vi "Autonomous Independent.vi"() -> ()   [LabVIEW 2019]
doc: "This VI is called when autonomous begins, and will automatically be terminated when autonomous ends. You can carry out timed or sensor driven robot movement independently without needing to return to the caller."
uses:
  Robot Global Data.vi
  <vilib>/Rock Robotics/Network Tables/SD Write Boolean.vi
panel:
  in  "v scale":dbl=1.0
  # "Be sure to right-click and choose Data Operations>>Make Current Value default if you want to save the array values with the VI"
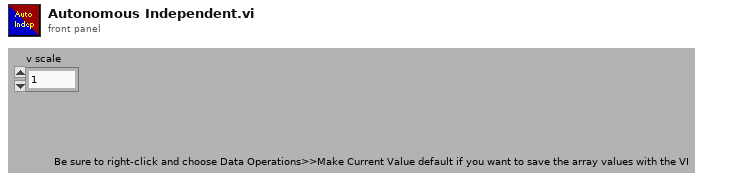
[diagram p1: front panel]
types:
  T1 = typedef "WPI_JoystickDevRef.ctl" = cluster{"Device":T2}
  T2 = typedef "WPI_JoystickDeviceEnum.ctl" = enum16{"USB 0", "USB 1", "USB 2", "USB 3", "USB 4", "USB 5"}
  T3 = cluster{"Cluster":cluster{"Path Backwards":bool, "Robot Backwards":bool}, "Traj Vel Points":cluster{"V":dbl, "th":dbl}[], cluster{"Sample Period (s)":dbl, cluster{"Velocity (fps)":dbl, "Acceleration (fps^2)":dbl, "Jerk (fps^3)":dbl, dbl}, "Conditions":cluster{"vInitial (fps)":dbl, "vFinal (fps)":dbl}, "Angular Accelerations":cluster{"Angular \nAccelerations":dbl[], "Override Limits?":bool[]}}}[]
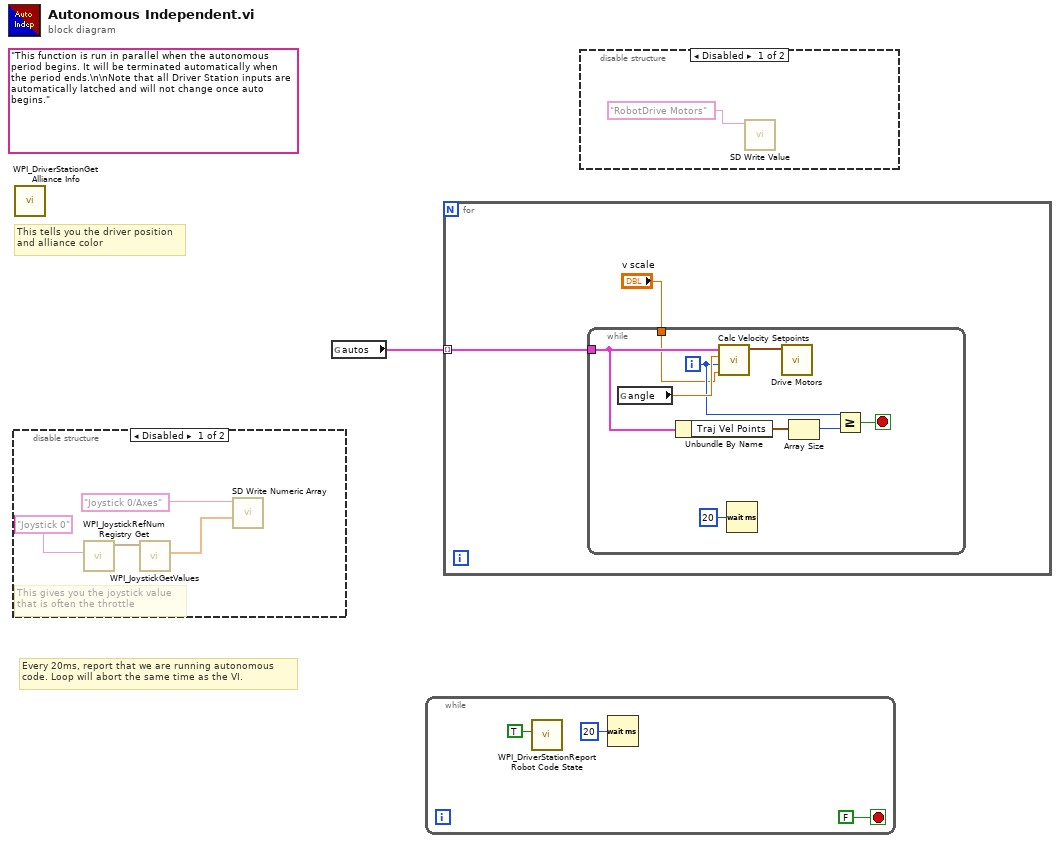
[diagram p0: block diagram]
diagram:
  (unwired) "This function is run in parallel when the autonomous period begins. It will be terminated automatically when the period ends.\n\nNote that all Driver Station inputs are automatically latched and will not change once auto begins."
  # "Every 20ms, report that we are running autonomous\ncode. Loop will abort the same time as the VI."
  # "This tells you the driver position\nand alliance color"
  n1 = disable-structure shown="Disabled" {
    frame Disabled {
      # "This gives you the joystick value\nthat is often the throttle"
      n2 = call <vilib>:"WPI_JoystickRefNum Registry Get.vi"("refnum name"="Joystick 0") -> ("JoystickDevRef"=w4:T1)  [unwired: 1 in, 9 out]
      n3 = call <vilib>:"WPI_JoystickGetValues.vi"("JoystickDevRef"=w4) -> ("Axes"=w2:dbl[])  [unwired: 6 in, 4 out]
      n4 = call <vilib>:"SD Write Numeric Array.vi"("Numeric Array"=w2, "Name"="Joystick 0/Axes") -> ()  [unwired: 8 in, 2 out]
    }
    frame Enabled {
    }
  }
  n5 = call <vilib>:"WPI_DriverStationGet Alliance Info.vi"() -> ()  [unwired: 12 out]
  n6 = global read "Robot Global Data.vi" "autos"() -> (w1:T3)
  n7 = while {
    stop <- FALSE stop-if-true
    n8 = call <vilib>:"WPI_DriverStationReport Robot Code State.vi"("Autonomous"=TRUE) -> ()  [unwired: 10 in, 1 out]
    n9 = Wait (ms)(milliseconds to wait=u32 20) -> ()  [unwired: 1 out]
  }
  n10 = for {
    tunnel: w1 -> [w10] mode=indexing
    n11 = while {
      tunnel: w10 -> [w16]
      tunnel: "v scale" -> [w11]
      i -> [w13]
      stop <- w12 stop-if-true
      n12 = global read "Robot Global Data.vi" "angle"() -> (w18:dbl)
      n13 = Unbundle By Name(w16) -> ("Traj Vel Points"=w15:cluster{"V":dbl, "th":dbl}[])
      n14 = call "Calc Velocity Setpoints.vi"("v scale"=w11, "Iterations"=w13, "Angle"=w18, "Path stuff"=w16) -> ("setpoints"=w17:cluster{"left":dbl, "right":dbl})  [unwired: 7 in]
      n15 = Wait (ms)(milliseconds to wait=u32 20) -> ()  [unwired: 1 out]
      n16 = call "Drive Motors.vi"("Cluster"=w17) -> ()  [unwired: 9 in, 2 out]
      n17 = Array Size(array=w15) -> (size(s)=w14:i32)
      n18 = Greater Or Equal?(x=w13, y=w14) -> (x >= y?=w12:bool)
    }
  }
  n19 = disable-structure shown="Disabled" {
    frame Disabled {
      n20 = call-poly <vilib>:"SD Write Value.vi"("Name"="RobotDrive Motors") -> ()  [unwired: 9 in, 2 out]
    }
    frame Enabled {
    }
  }
